vi "Load Simulation.vi"(0 "reference in":refnum<class "Battery.lvclass">, 2 "Simulation Parameters":T1={"# RC Pairs"=1, "R0 (Ohm)"=0.0015, "R1 (Ohm)"=0.001, "C1 (Farad)"=2500.0, "R2 (Ohm)"=0.0008, "C2 (Farad)"=40000.0, "Nominal Capacity (Ah)"=5.0, "Upper Cutoff Voltage"=4.2, "Lower Cutoff Voltage"=3.0, "Coulombic Efficiency"=3.0} {"# RC Pairs" min=1 max=2}, 5 "Error In":errorcluster) -> (14 "reference out":refnum<class "Battery.lvclass">, 16 "simulation loaded":bool, 19 "Error Out":errorcluster)   [LabVIEW 2023, in "Battery.lvclass"]
uses:
  Battery.lvclass
  Simulation Parameters.ctl
  Battery.lvclass/Battery.ctl
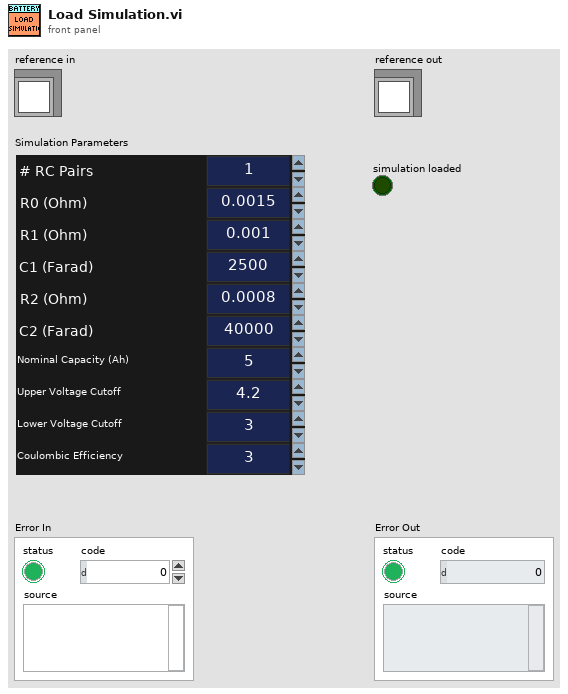
[diagram p1: front panel]
types:
  T1 = typedef "Battery.lvclass/Simulation Parameters.ctl" = cluster{"# RC Pairs":u8, "R0 (Ohm)":dbl, "R1 (Ohm)":dbl, "C1 (Farad)":dbl, "R2 (Ohm)":dbl, "C2 (Farad)":dbl, "Nominal Capacity (Ah)":dbl, "Upper Cutoff Voltage":dbl, "Lower Cutoff Voltage":dbl, "Coulombic Efficiency":dbl}
  T2 = typedef "Battery.lvclass/ObjectAttributes.ctl" = cluster{"Python module":path, "Python Session":refnum<k35>, "PybammWrapper":refnum<k38>, "simulation loaded":bool, "simulation enabled":bool, "SOC OCV Curve":dbl[][], "Open Circuit Voltage (V)":dbl, "Terminal Voltage (V)":dbl, "State of Charge (%)":dbl, "# Cells in Series":u16, "# Cells in Parallel":u16, "Simulation Parameters":T1, "Power Module":refnum<class "PowerModuleInterface.lvclass">}
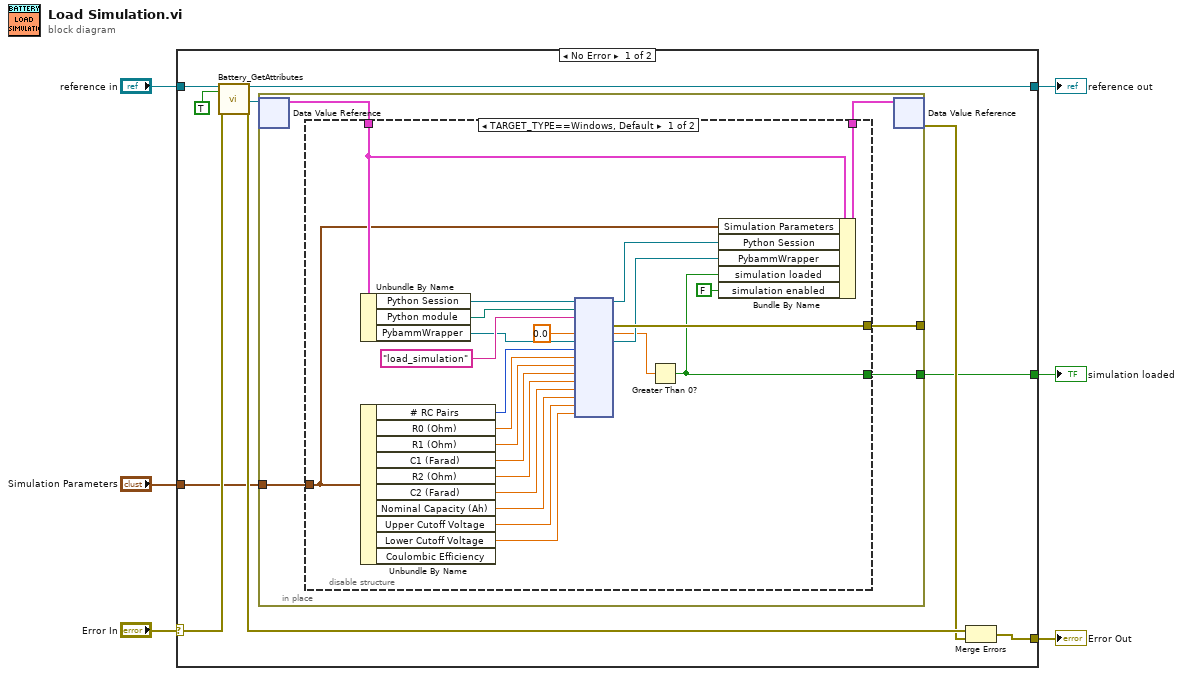
[diagram p0: block diagram]
diagram:
  n1 = case shown="No Error" "Error In" {
    selector: "Error In" -> [w15 w47]
    tunnel: [w13 w47] -> w5
    tunnel: [w14 w46] -> w3
    tunnel: "reference in" -> [w16 w46]
    tunnel: "Simulation Parameters" -> [w8 _]
    tunnel: [w7 _] -> w1
    frame No Error {
      n2 = call "Battery_GetAttributes.vi"("reference in"=w16, "OnlyGetDvrReference(False)"=TRUE, "Error In"=w15) -> ("reference out"=w14:refnum<class "Battery.lvclass">, "DataRef"=w12:refnum<data-value>, "Error Out"=w10:errorcluster)  [unwired: 13 in, 1 out]
      n3 = in-place {
        in-place-border: w8 -> [w17]
        in-place-border: [w19] -> _
        in-place-border: [w18] -> w7
        n4 = in-place-dvr #1(w12) -> (w20:T2)  [unwired: 1 out]
        n5 = disable-structure shown="TARGET_TYPE==Windows, Default" {
          disable-tunnel: [w44 w45] -> w21
          disable-tunnel: w20 -> [w43 w45]
          disable-tunnel: [w33 _] -> w19
          disable-tunnel: [w23 _] -> w18
          disable-tunnel: w17 -> [w28 _]
          frame condition #0 (active) {
            n6 = Unbundle By Name(w43) -> ("Python Session"=w30:refnum<k35>, "Python module"=w31:path, "PybammWrapper"=w32:refnum<k38>)
            n7 = Unbundle By Name(w28) -> ("# RC Pairs"=w41:u8, "R0 (Ohm)"=w40:dbl, "R1 (Ohm)"=w39:dbl, "C1 (Farad)"=w38:dbl, "R2 (Ohm)"=w37:dbl, "C2 (Farad)"=w36:dbl, "Nominal Capacity (Ah)"=w26:dbl, "Upper Cutoff Voltage"=w35:dbl, "Lower Cutoff Voltage"=w34:dbl)  [unwired: 1 out]
            n8 = node(w30, w31, "load_simulation" ("function name"), 0.0, w32, w41, w40, w39, w38, w37, w36, w26, w35, w34) -> (w27:refnum<k35>, w33:errorcluster, w24:dbl, w29:refnum<k38>)  [unwired: 10 in, 2 out]
            n9 = Greater Than 0?(x=w24) -> (x > 0?=w23:bool)
            n10 = Bundle By Name(cluster=w43, "Simulation Parameters"=w28, "Python Session"=w27, "PybammWrapper"=w29, "simulation loaded"=w23, "simulation enabled"=FALSE) -> (w44:T2)
          }
          frame condition #1 {
          }
        }
        n11 = in-place-dvr #1(w21) -> (w9:errorcluster)  [unwired: 1 out]
      }
      n12 = Merge Errors(w10, w9) -> (w13:errorcluster)
    }
    frame Error {
    }
  }
  "Error Out" <- w5
  "reference out" <- w3
  "simulation loaded" <- w1
